vi "Aperture.vi"(8 "error in (no error)":errorcluster, 9 "Averaging Rate (1)":i16=1 min=1 max=256 step=1, 10 "Integ Time (0: Short)":u32(slide) max=2 step=1, 11 "VISA resource name":refnum<visa-resource-name>) -> (0 "error out":errorcluster, 3 "VISA resource name out":refnum<visa-resource-name>)   [LabVIEW 2015, in "Agilent 428X Series.lvlib"]
doc: "The Aperture function sets the integration time of the A/D converter and the averaging rate."
uses:
  Agilent 428X Series.lvlib
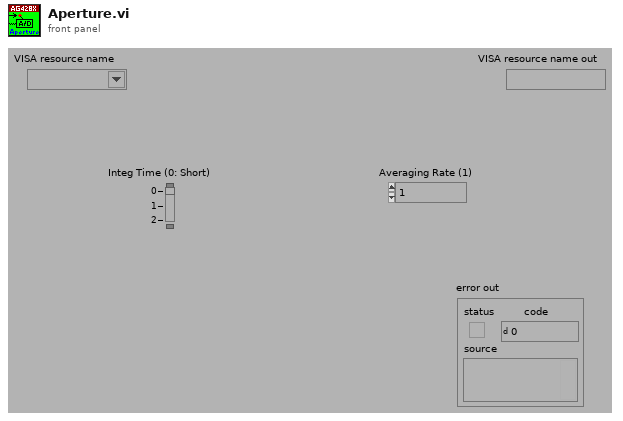
[diagram p1: front panel]
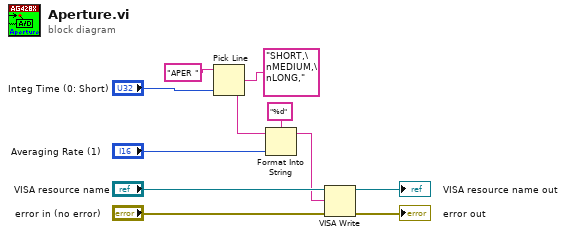
[diagram p0: block diagram]
diagram:
  n1 = Pick Line(string ("")="APER ", multi-line string="SHORT,\nMEDIUM,\nLONG,", line index="Integ Time (0: Short)") -> (output string=w3:string)
  n2 = Format Into String(format string="%d", initial string=w3, "Averaging Rate (1)") -> (resulting string=w1:string)  [unwired: 1 in, 1 out]
  n3 = VISA Write(VISA resource name="VISA resource name", write buffer=w1, error in (no error)="error in (no error)") -> (VISA resource name out=→"VISA resource name out":refnum<visa-resource-name>, error out=→"error out":errorcluster)  [unwired: 1 out]
